vi "FTW-JSON-Array-Elements.vi"(0 "JSON":T1, 11 "error in":errorcluster) -> (4 "JSON out":T1, 6 "Elements":string[](array[string]), 15 "error out":errorcluster)   [LabVIEW 2015]
uses:
  core/type/FTW-Type-JSON.ctl
panel:
  # "Inputs"
  # "Outputs"
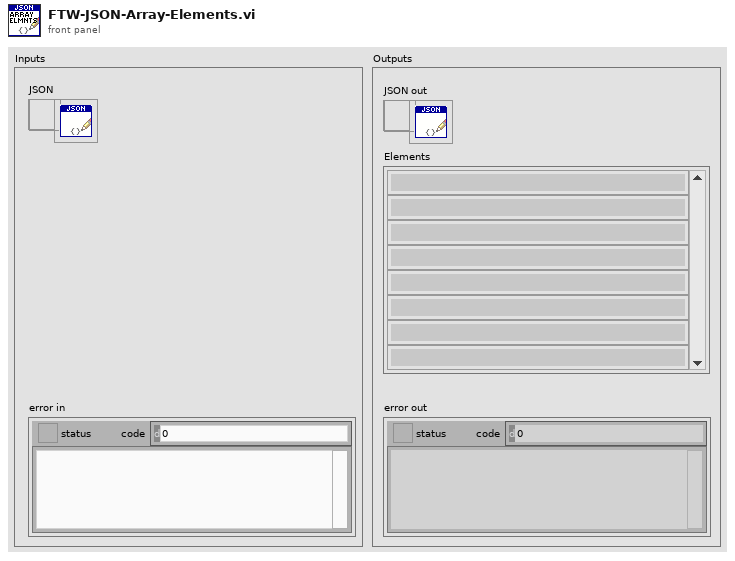
[diagram p1: front panel]
types:
  T1 = typedef "FTW-Type-JSON.ctl" = refnum<data-value>
  T2 = cluster{"FTW-CodeGen-Type":enum16{"FTW-JSON"}, "Object":i64, "EncodingFlags":i64, "DecodingFlags":i64}
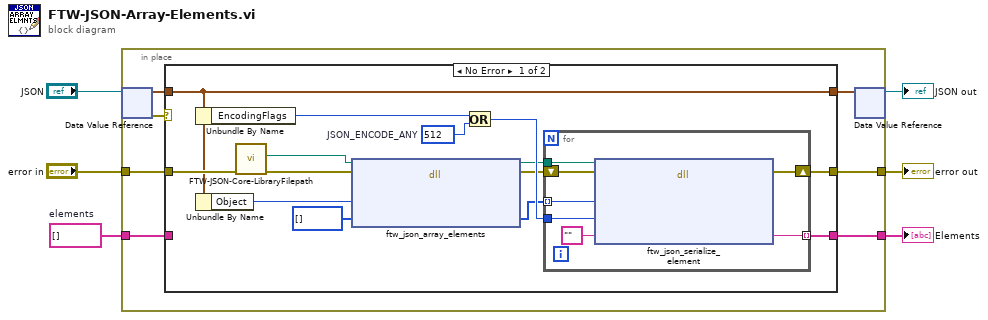
[diagram p0: block diagram]
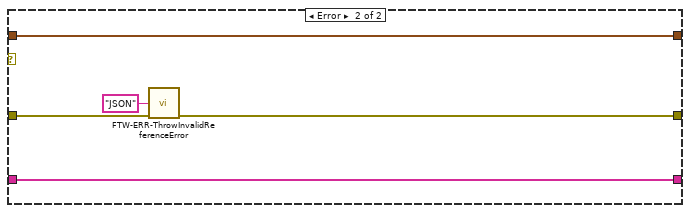
[diagram p2: hidden frame]
diagram:
  w1 = string[] []  # elements
  n1 = in-place {
    in-place-border: [w10] -> w6
    in-place-border: [w11] -> w2
    in-place-border: "error in" -> [w9]
    in-place-border: w1 -> [w12]
    n2 = in-place-dvr #1("JSON") -> (w13:T2, w7:errorcluster)
    n3 = case shown="No Error" w7 {
      tunnel: w13 -> [w17 w39]
      tunnel: w12 -> [_ w35]
      tunnel: [w14 w35] -> w11
      tunnel: [w18 w36] -> w10
      tunnel: w9 -> [w27 w37]
      tunnel: [w17 w39] -> w8
      frame No Error {
        w21 = i64 512  # JSON_ENCODE_ANY
        n4 = Unbundle By Name(w17) -> ("EncodingFlags"=w16:i64)
        n5 = Unbundle By Name(w17) -> ("Object"=w23:i64)
        n6 = call "FTW-JSON-Core-LibraryFilepath.vi"("error in"=w27) -> ("error out"=w25:errorcluster, "JSON Library Filepath"=w24:path)  [unwired: 9 in]
        n7 = dll-call lib="?" fn="ftw_json_array_elements"(path in=w24, error in=w25, "Array Pointer"=w23, "Items"=i64[] []) -> (path out=w20:path, error out=w19:errorcluster, "Items"=w15:i64[])  [unwired: 3 in]
        n8 = Or(x=w16, y=w21) -> (x .or. y?=w22:i64)
        n9 = for {
          tunnel: w22 -> [w34]
          tunnel: w20 -> [w33]
          shift-right: [w31] -> w18
          shift-left: w19 -> [w32]
          tunnel: w15 -> [w29] mode=indexing
          tunnel: [w28] -> w14 mode=indexing
          n10 = dll-call lib="?" fn="ftw_json_serialize_element"(path in=w33, error in=w32, "JSON Object Pointer"=w29, "Flags"=w34, "Serialized String"="" ("empty string")) -> (error out=w31:errorcluster, "Serialized String"=w28:string)  [unwired: 4 in, 1 out]
        }
      }
      frame Error {
        n11 = call "FTW-ERR-ThrowInvalidReferenceError.vi"("Reference Type"="JSON", "error in"=w37) -> ("error out"=w36:errorcluster)  [unwired: 13 in]
      }
    }
    n12 = in-place-dvr #1(w8) -> (→"JSON out":T1)  [unwired: 1 out]
  }
  "error out" <- w6
  "Elements" <- w2
